vi "Determine if Mouse is in Bounds.vi"(9 "Coords":T1, 11 "XYGraph in":refnum<vi>) -> (3 "In bounds?":bool)   [LabVIEW 2015]
uses:
  <vilib>/Utility/miscctls.llb/LVPoint32TypeDef.ctl
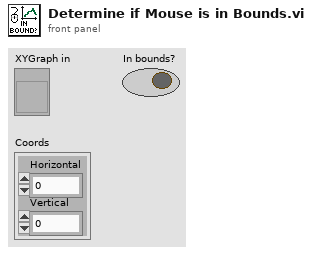
[diagram p1: front panel]
types:
  T1 = typedef "LVPoint32TypeDef.ctl" = cluster{"Horizontal":i32, "Vertical":i32}
  T2 = typedef "LVRectTypeDef.ctl" = cluster{"Left":i16, "Top":i16, "Right":i16, "Bottom":i16}
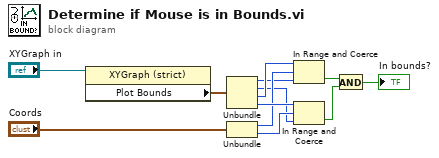
[diagram p0: block diagram]
diagram:
  n1 = property on="Property Node" class="XYGraph (strict)"(reference="XYGraph in") -> ("Plot Bounds"=w1:T2)  [unwired: 1 in, 2 out]
  n2 = Unbundle(w1) -> ("Left"=w2:i16, "Top"=w3:i16, "Right"=w6:i16, "Bottom"=w7:i16)
  n3 = Unbundle("Coords") -> ("Horizontal"=w5:i32, "Vertical"=w4:i32)
  n4 = In Range and Coerce(upper limit=w6, x=w5, lower limit=w2) -> (In Range?=w8:bool)  [unwired: 1 out]
  n5 = In Range and Coerce(upper limit=w7, x=w4, lower limit=w3) -> (In Range?=w9:bool)  [unwired: 1 out]
  n6 = And(x=w8, y=w9) -> (x .and. y?=→"In bounds?":bool)
